vi "Periodic Tasks.vi"(8 "error in":errorcluster) -> ()   [LabVIEW 2020]
doc: "This VI runs in parallel to other tasks. It can contain as many user-defined periodic loops as you need. These can carry out PID or other sorts of timed response."
uses:
  Globals/Turret_Globals.vi
  <vilib>/Rock Robotics/Network Tables/NT Write Boolean.vi
  Globals/Flywheel_Globals.vi
  Globals/Calibration_And_Constant_Globals.vi
  Globals/Cowl_Globals.vi
panel:
  # "eeeeeeeeeeeeeeeeeee"
  # "eeeeeeeeeeeeeeeeeeee"
  # "eeeeeeeeeee"
  # "eeeeeeeeeeeeeeeeeeee"
  # "eeeeeeeeeee"
  # "eeeeeeeeeee"
  # "eeee"
  # "eeeeeeeeeee"
  # "e"
  # "e"
  # "e"
  # "e"
  # "e"
  # "e"
  # "e"
  # "eeeeeeeeeeeeeeeeeee"
  # "e"
  # "e"
  # "e"
  # "e"
  # "e"
  # "e"
  # "e"
  # "e"
  # "e"
  # "e"
  # "e"
  # "e"
  # "e"
  # "e"
  # "e"
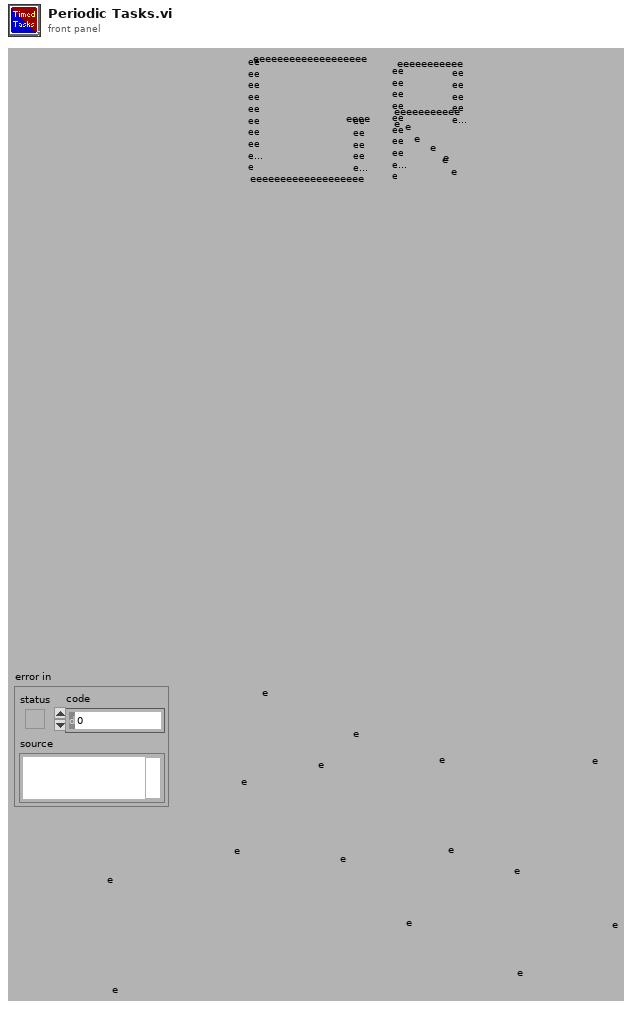
[diagram p1: front panel]
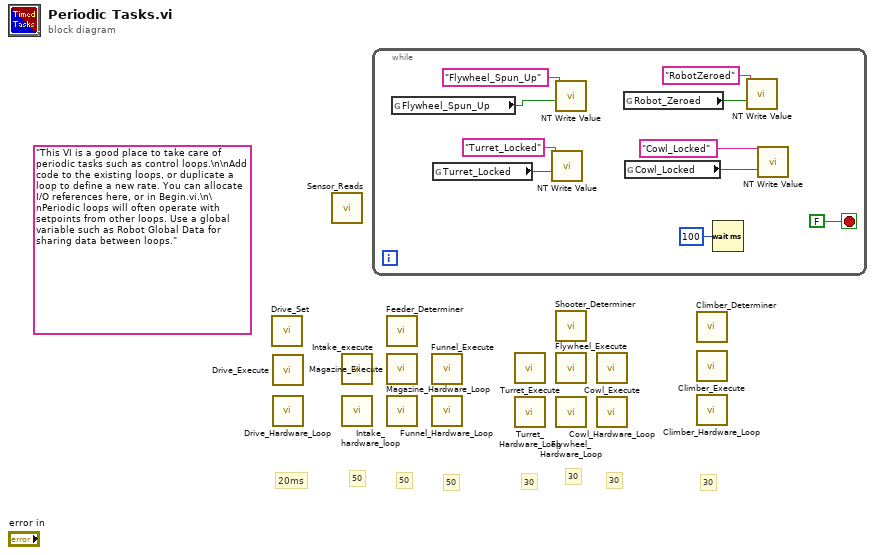
[diagram p0: block diagram]
diagram:
  (unwired) "This VI is a good place to take care of periodic tasks such as control loops.\n\nAdd code to the existing loops, or duplicate a loop to define a new rate. You can allocate I/O references here, or in Begin.vi.\n\nPeriodic loops will often operate with setpoints from other loops. Use a global variable such as Robot Global Data for sharing data between loops."
  # "30"
  # "30"
  # "30"
  # "30"
  # "50"
  # "50"
  # "50"
  # "20ms"
  n1 = call "Drive_Set.vi"() -> ()  [unwired: 12 in]
  n2 = call "Drive_Execute.vi"() -> ()  [unwired: 12 in]
  n3 = call "Drive_Hardware_Loop.vi"() -> ()  [unwired: 12 in]
  n4 = call "Sensor_Reads.vi"() -> ()  [unwired: 12 in]
  n5 = call "Intake_execute.vi"() -> ()  [unwired: 12 in]
  n6 = call "Intake_hardware_loop.vi"() -> ()  [unwired: 12 in]
  n7 = while {
    stop <- FALSE stop-if-true
    n8 = global read "Flywheel_Globals.vi" "Flywheel_Spun_Up"() -> (w6:bool)
    n9 = global read "Turret_Globals.vi" "Turret_Locked"() -> (w7:bool)
    n10 = call-poly <vilib>:"NT Write Value.vi"("Boolean"=w7, "Name"="Turret_Locked") -> ()  [unwired: 9 in, 1 out]
    n11 = call-poly <vilib>:"NT Write Value.vi"("Boolean"=w6, "Name"="Flywheel_Spun_Up") -> ()  [unwired: 9 in, 1 out]
    n12 = global read "Calibration_And_Constant_Globals.vi" "Robot_Zeroed"() -> (w5:bool)
    n13 = global read "Cowl_Globals.vi" "Cowl_Locked"() -> (w4:bool)
    n14 = Wait (ms)(milliseconds to wait=u32 100) -> ()  [unwired: 1 out]
    n15 = call-poly <vilib>:"NT Write Value.vi"("Boolean"=w5, "Name"="RobotZeroed") -> ()  [unwired: 9 in, 1 out]
    n16 = call-poly <vilib>:"NT Write Value.vi"("Boolean"=w4, "Name"="Cowl_Locked") -> ()  [unwired: 9 in, 1 out]
  }
  n17 = call "Feeder_Determiner.vi"() -> ()  [unwired: 12 in]
  n18 = call "Magazine_Execute.vi"() -> ()  [unwired: 12 in]
  n19 = call "Magazine_Hardware_Loop.vi"() -> ()  [unwired: 12 in]
  n20 = call "Funnel_Execute.vi"() -> ()  [unwired: 12 in]
  n21 = call "Funnel_Hardware_Loop.vi"() -> ()  [unwired: 12 in]
  n22 = call "Turret_Execute.vi"() -> ()  [unwired: 12 in]
  n23 = call "Turret_Hardware_Loop.vi"() -> ()  [unwired: 12 in]
  n24 = call "Shooter_Determiner.vi"() -> ()  [unwired: 12 in]
  n25 = call "Flywheel_Execute.vi"() -> ()  [unwired: 12 in]
  n26 = call "Flywheel_Hardware_Loop.vi"() -> ()  [unwired: 12 in]
  n27 = call "Cowl_Execute.vi"() -> ()  [unwired: 12 in]
  n28 = call "Cowl_Hardware_Loop.vi"() -> ()  [unwired: 12 in]
  n29 = call "Climber_Determiner.vi"() -> ()  [unwired: 12 in]
  n30 = call "Climber_Execute.vi"() -> ()  [unwired: 12 in]
  n31 = call "Climber_Hardware_Loop.vi"() -> ()  [unwired: 12 in]
